vi "XY bar graph(1) .vi"() -> ()   [LabVIEW 2014]
panel:
  out "XY Graph":cluster{"X-axis":dbl[], "Y-axis":dbl[]}(graph)
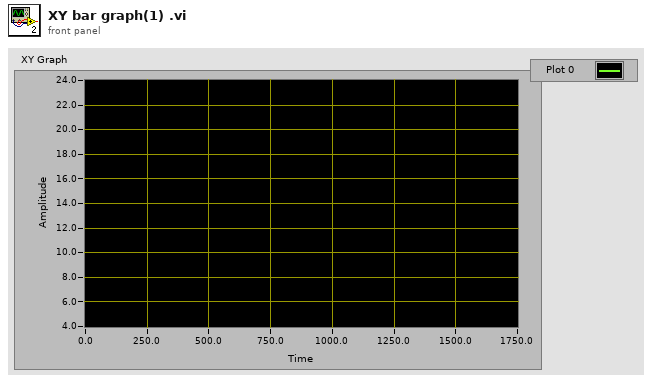
[diagram p1: front panel]
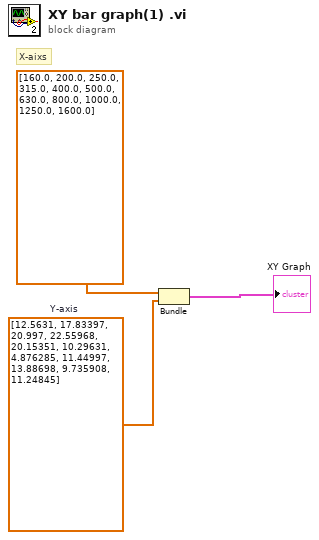
[diagram p0: block diagram]
diagram:
  w3 = dbl[] [12.5631, 17.83397, 20.997, 22.55968, 20.15351, 10.29631, 4.876285, 11.44997, 13.88698, 9.735908, 11.24845]  # Y-axis
  # "X-aixs"
  n1 = Bundle("X-axis"=dbl[] [160.0, 200.0, 250.0, 315.0, 400.0, 500.0, 630.0, 800.0, 1000.0, 1250.0, 1600.0], "Y-axis"=w3) -> (→"XY Graph":cluster{"X-axis":dbl[], "Y-axis":dbl[]})  [unwired: 1 in]
